vi "LabVIEW 2.vi"() -> ()   [LabVIEW 2024]
panel:
  in  "Keep Prev Locations":bool
  in  "stop":bool
  out "2D Picture":picture
  # "Christian Belga\nSE 423\n2/27/25"
  # "255.255.255.0"
  # "Ethernet adapter Ethernet 2:\n\n   Connection-specific DNS Suffix  . :\n   IPv6 Address. . . . . . . . . . . : 2620:0:e00:4037::14a\n   Link-local IPv6 Address . . . . . : fe80::1277:6ca6:a9c4:4798%3\n   IPv4 Address. . . . . . . . . . . : 10.251.132.221\n   Subnet Mask . . . . . . . . . . . : 255.255.240.0\n   Default Gateway . . . . . . . . . :\n\nEthernet adapter Ethernet:\n\n   Connection-specific DNS Suffix  . :\n   Link-local IPv6 Address . . . . . : fe80::a820:4e3a:f3c4:4c2d%9\n   IPv4 Address. . . . . . . . . . . : 173.230.99.63\n   Subnet Mask . . . . . . . . . . . : 255.255.255.0\n   Default Gateway . . . . . . . . . : 173.230.99.1"
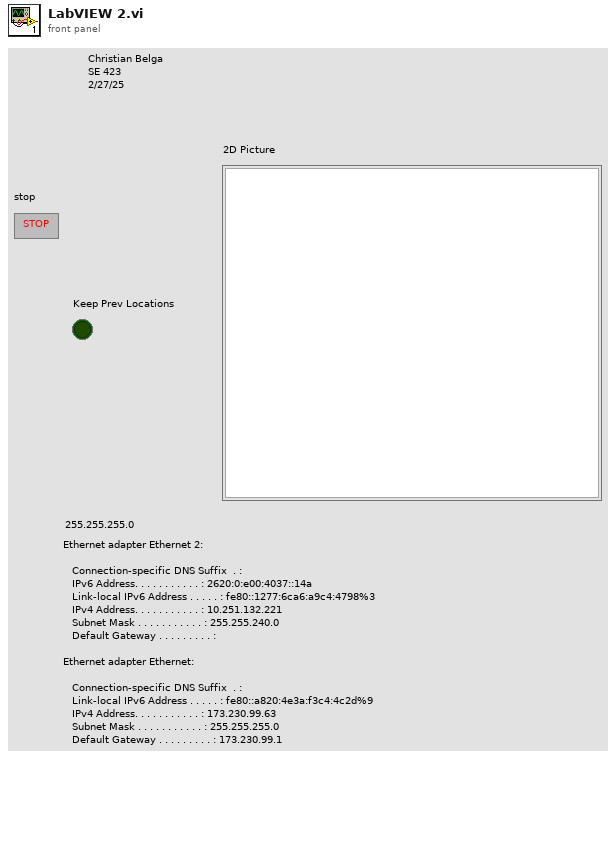
[diagram p1: front panel]
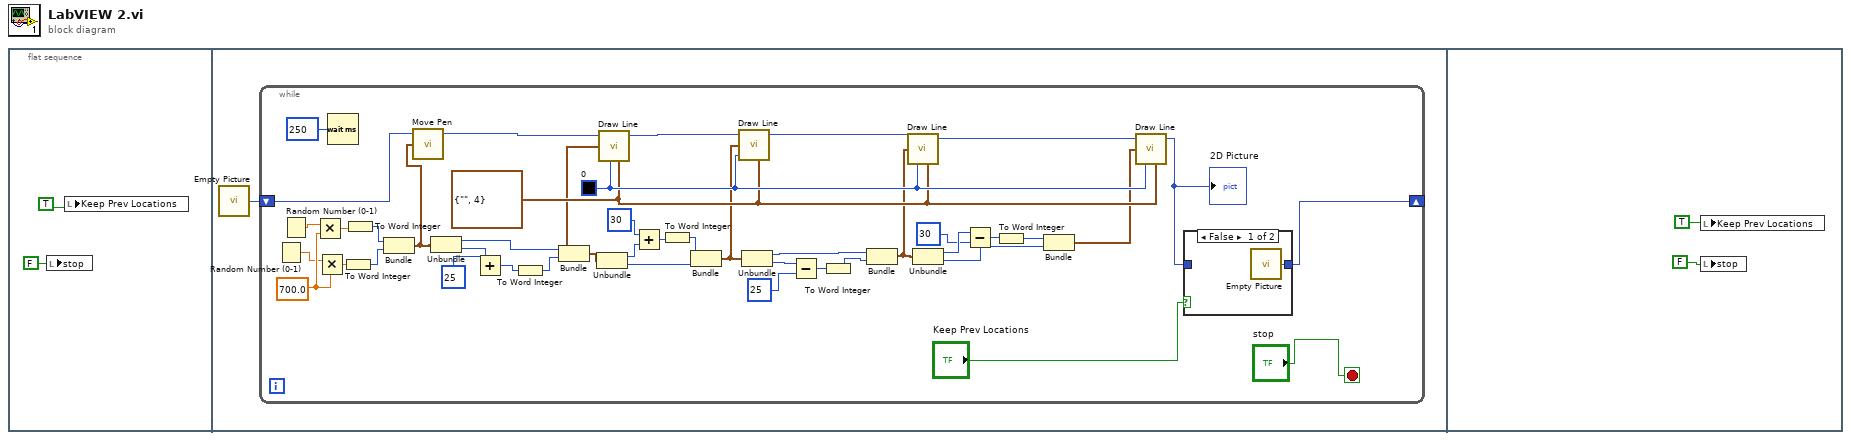
[diagram p0: block diagram]
diagram:
  n1 = flat-sequence {
    frame #0 {
      n2 = local write "stop"(FALSE) -> ()
      n3 = local write "Keep Prev Locations"(TRUE) -> ()
    }
    frame #1 {
      n4 = call "Empty Picture"() -> ("empty picture"=w3:picture)
      n5 = while {
        shift-right: [w6] -> _
        shift-left: w3 -> [w46]
        stop <- "stop" stop-if-true
        w28 = u32 0
        w27 = cluster{enum16{""}, i32} {enum."", 4}
        w40 = 700.0 ("y")
        n6 = Random Number (0-1)() -> (number: 0 to 1=w39:dbl)
        n7 = Random Number (0-1)() -> (number: 0 to 1=w38:dbl)
        n8 = Multiply(x=w38, y=w40) -> (x*y=w37:dbl)
        n9 = Multiply(x=w39, y=w40) -> (x*y=w36:dbl)
        n10 = Wait (ms)(milliseconds to wait=u32 250) -> ()  [unwired: 1 out]
        n11 = To Word Integer(number=w36) -> (16bit integer=w35:i16)
        n12 = To Word Integer(number=w37) -> (16bit integer=w34:i16)
        n13 = Bundle(w34, w35) -> (w33:cluster{i16, i16})  [unwired: 1 in]
        n14 = call <vilib>:"Move Pen.vi"("new position"=w33, "picture"=w46) -> ("new picture"=w45:picture)  [unwired: 3 in]
        n15 = Unbundle(w33) -> (w29:i16, w32:i16)
        n16 = Add(x=w32, y=i16 25) -> (x+y=w30:i16)
        n17 = To Word Integer(number=w30) -> (16bit integer=w23:i16)
        n18 = Bundle(w29, w23) -> (w24:cluster{i16, i16})  [unwired: 1 in]
        n19 = Unbundle(w24) -> (w20:i16, w22:i16)
        n20 = call <vilib>:"Draw Line.vi"("picture"=w45, "end point"=w24, "color(black)"=w28, "pen"=w27) -> ("new picture"=w44:picture)  [unwired: 5 in]
        n21 = Add(x=i16 30 ("y"), y=w20) -> (x+y=w25:i16)
        n22 = To Word Integer(number=w25) -> (16bit integer=w21:i16)
        n23 = Bundle(w21, w22) -> (w19:cluster{i16, i16})  [unwired: 1 in]
        n24 = call <vilib>:"Draw Line.vi"("picture"=w44, "end point"=w19, "color(black)"=w28, "pen"=w27) -> ("new picture"=w43:picture)  [unwired: 5 in]
        n25 = Unbundle(w19) -> (w15:i16, w18:i16)
        n26 = Subtract(x=w18, y=i16 25) -> (x-y=w16:i16)
        n27 = To Word Integer(number=w16) -> (16bit integer=w14:i16)
        n28 = Bundle(w15, w14) -> (w12:cluster{i16, i16})  [unwired: 1 in]
        n29 = call <vilib>:"Draw Line.vi"("picture"=w43, "end point"=w12, "color(black)"=w28, "pen"=w27) -> ("new picture"=w42:picture)  [unwired: 5 in]
        n30 = Unbundle(w12) -> (w13:i16, w10:i16)
        n31 = Subtract(x=w13, y=i16 30) -> (x-y=w9:i16)
        n32 = To Word Integer(number=w9) -> (16bit integer=w8:i16)
        n33 = Bundle(w8, w10) -> (w7:cluster{i16, i16})  [unwired: 1 in]
        n34 = call <vilib>:"Draw Line.vi"("picture"=w42, "end point"=w7, "color(black)"=w28, "pen"=w27) -> ("new picture"=w41:picture)  [unwired: 5 in]
        "2D Picture" <- w41
        n35 = case shown="False" "Keep Prev Locations" {
          tunnel: [w48 w49] -> w6
          tunnel: w41 -> [_ w49]
          frame False {
            n36 = call "Empty Picture"() -> ("empty picture"=w48:picture)
          }
          frame True {
          }
        }
      }
    }
    frame #2 {
      n37 = local write "Keep Prev Locations"(TRUE) -> ()
      n38 = local write "stop"(FALSE) -> ()
    }
  }
